vi "error.get_last.vi"(8 "error in (no error)":errorcluster, 10 "buf_len":i32, 11 "buf_ptr":string) -> (0 "error out":errorcluster, 2 "function return":i32, 3 "buf_ptr out":string)   [LabVIEW 2020, in "reqwest-labview.lvlib"]
doc: "Retrieves a human-readable description of the last error that occurred on the calling thread.\n\n\n\n\n\n\nint http_get_last_error(unsigned char *buf_ptr,\n int buf_len);"
uses:
  reqwest-labview.lvlib
  http_rs_labview.dll
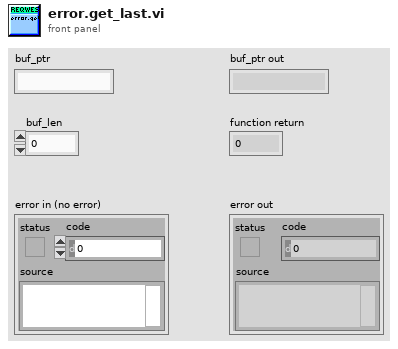
[diagram p1: front panel]
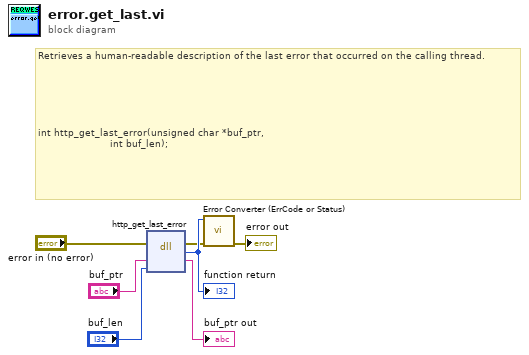
[diagram p0: block diagram]
diagram:
  # "Retrieves a human-readable description of the last error that occurred on the calling thread.\n\n\n\n\n\n\nint http_get_last_error(unsigned char *buf_ptr,\n                        int buf_len);"
  n1 = dll-call lib="C:/code/reqwest-labview/lv-src/shared-library/http_rs_labview.*" fn="http_get_last_error"(error in="error in (no error)", "buf_ptr"="buf_ptr", "buf_len"="buf_len") -> (error out=w2:errorcluster, w7:i32, "buf_ptr"=→"buf_ptr out":string)  [unwired: 3 in, 1 out]
  "function return" <- w7
  n2 = call "Error Converter (ErrCode or Status).vi"("error in (no error)"=w2, "error code"=w7) -> ("error out"=→"error out":errorcluster)  [unwired: 9 in]
